vi "plot_radar_target_by_name.vi"(4 "error in":errorcluster={"status"=FALSE, "code"=0, "source"="Event Code: 0\r\ncomplete\r\n-----------------------------------\nEvent Code: 0\r\ncomplete\r\n-----------------------------------\nEvent Code: 0\r\nweather configured to \"Default\"\r\n-----------------------------------\nEvent Code: 0\r\ncomplete\r\n-----------------------------------\nEvent Code: 0\r\nsimulator configuration mode = 1\r\n-----------------------------------\nEvent Code: 0\r\nsimulator_version: 1.10.0, api_version: 3.0\r\n-----------------------------------\nEvent Code: 0\r\n\r\n-----------------------------------\n"}, 6 "Target id to track":string="compact_monoDrive_01_2", 7 "Radar Sample":T1={"Number of targets"=14, "gt_targets"=[], "target_list"=[{"aoa"=14.62, "range"=9.3, "rcs"=-11.41, "velocity"=-6.5, "target_ids"=["GuardRails14", "GuardRails13"]}, {"aoa"=-1.91, "range"=10.92, "rcs"=-12.49, "velocity"=-6.62, "target_ids"=[]}, {"aoa"=-1.49, "range"=12.13, "rcs"=-17.08, "velocity"=-6.5699997, "target_ids"=["truck_monoDrive_01_2"]}, {"aoa"=10.91, "range"=13.75, "rcs"=-16.51, "velocity"=-6.6499996, "target_ids"=["GuardRails14"]}, {"aoa"=9.55, "range"=14.549999, "rcs"=-14.82, "velocity"=-6.6499996, "target_ids"=["GuardRails14"]}, {"aoa"=8.45, "range"=16.17, "rcs"=-14.36, "velocity"=-6.64, "target_ids"=["GuardRails14"]}, {"aoa"=8.429999, "range"=17.789999, "rcs"=-10.95, "velocity"=-6.6499996, "target_ids"=["GuardRails14"]}, {"aoa"=6.6499996, "range"=20.21, "rcs"=-9.48, "velocity"=-6.64, "target_ids"=["GuardRails14"]}, {"aoa"=6.33, "range"=24.26, "rcs"=-13.74, "velocity"=-6.64, "target_ids"=["GuardRails15"]}, {"aoa"=13.61, "range"=27.09, "rcs"=-7.4199996, "velocity"=-6.6499996, "target_ids"=["InstancedFoliageActor_0"]}, {"aoa"=4.69, "range"=31.539999, "rcs"=-13.62, "velocity"=-6.64, "target_ids"=["GuardRails15"]}, {"aoa"=4.2999997, "range"=35.17, "rcs"=-11.82, "velocity"=-6.64, "target_ids"=["GuardRails15"]}, {"aoa"=-12.49, "range"=52.559998, "rcs"=12.82, "velocity"=-6.6499996, "target_ids"=["prp_electricalBox_142"]}, {"aoa"=-11.08, "range"=52.559998, "rcs"=12.82, "velocity"=-6.6499996, "target_ids"=["HighwaySign_30"]}], "tracks"=[], "roi_targets"=[]}) -> (0 "error out":errorcluster={"status"=FALSE, "code"=0, "source"="Event Code: 0\r\ncomplete\r\n-----------------------------------\nEvent Code: 0\r\ncomplete\r\n-----------------------------------\nEvent Code: 0\r\nweather configured to \"Default\"\r\n-----------------------------------\nEvent Code: 0\r\ncomplete\r\n-----------------------------------\nEvent Code: 0\r\nsimulator configuration mode = 1\r\n-----------------------------------\nEvent Code: 0\r\nsimulator_version: 1.10.0, api_version: 3.0\r\n-----------------------------------\nEvent Code: 0\r\n\r\n-----------------------------------\n"})   [LabVIEW 2019, in "Lib_Simx.lvlib"]
doc: "Tool generates a plot to compare AoA, Range and Velocity between the GT targets and the target list from the Radar sensor. This tool only tracks one target by the specified target on the Name of Target control."
uses:
  Lib_Simx.lvlib
  controls/radarSample.ctl
  controls/RadarTrack.ctl
panel:
  out "Velocity":cluster{"t":sgl, "t":sgl}(graph)
  out "Range":cluster{"t":sgl, "t":sgl}(graph)
  out "Aoa":cluster{"t":sgl, "t":sgl}(graph)
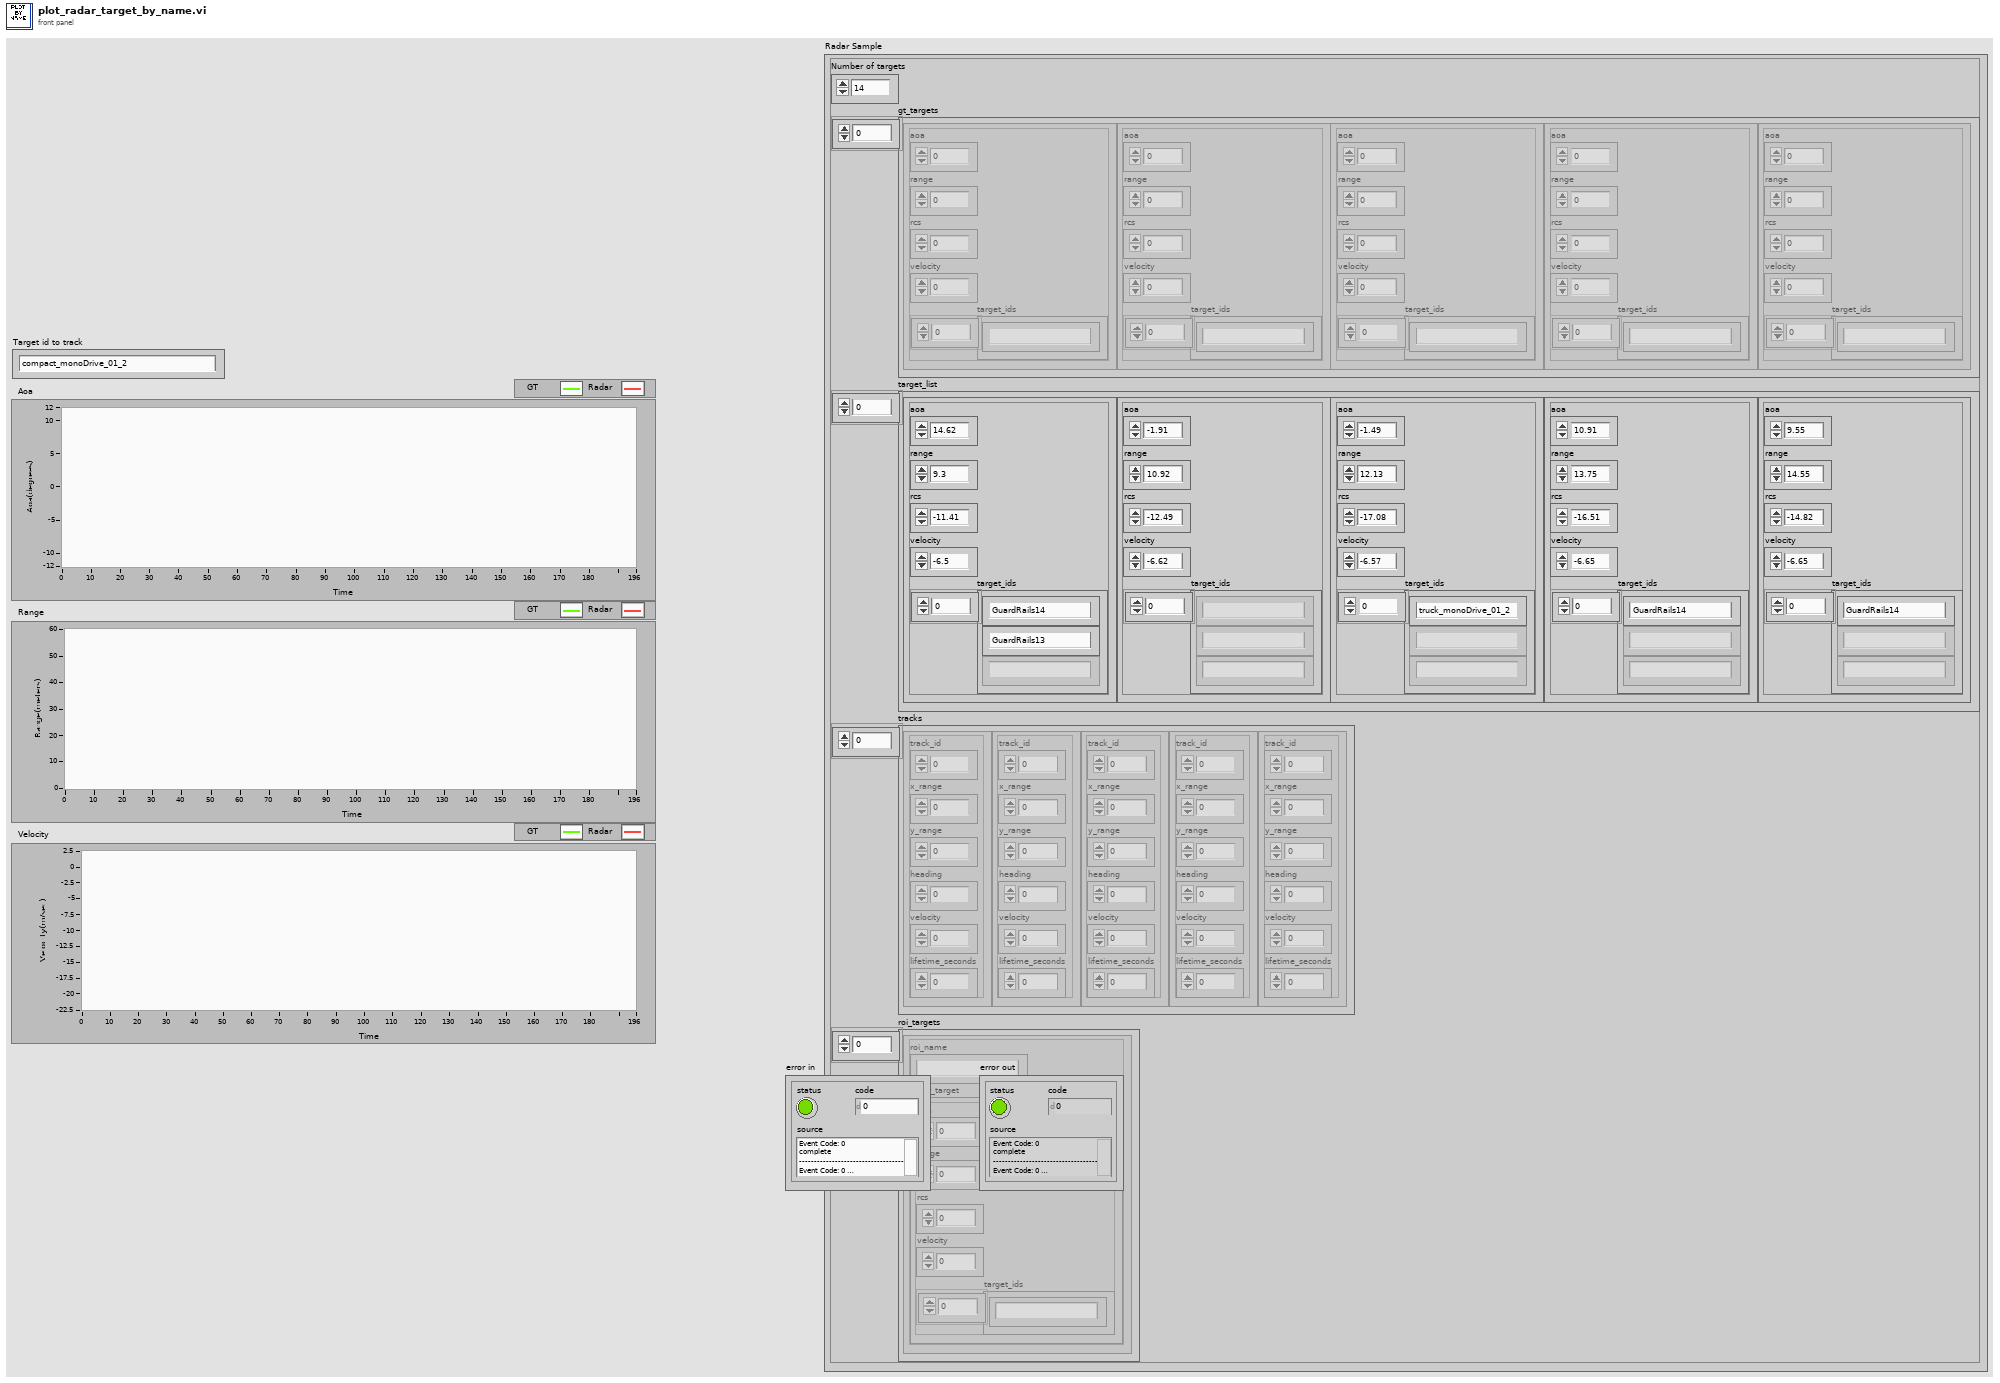
[diagram p1: front panel]
types:
  T1 = typedef "Lib_Simx.lvlib/radarSample.ctl" = cluster{"Number of targets":i32, "gt_targets":cluster{"aoa":sgl, "range":sgl, "rcs":sgl, "velocity":sgl, "target_ids":string[]}[], "target_list":cluster{"aoa":sgl, "range":sgl, "rcs":sgl, "velocity":sgl, "target_ids":string[]}[], "tracks":T2[], "roi_targets":cluster{"roi_name":string, "radar_target":cluster{"aoa":sgl, "range":sgl, "rcs":sgl, "velocity":sgl, "target_ids":string[]}}[]}
  T2 = typedef "Lib_Simx.lvlib/RadarTrack.ctl" = cluster{"track_id":u64, "x_range":sgl, "y_range":sgl, "heading":sgl, "velocity":sgl, "lifetime_seconds":sgl}
  T3 = cluster{"aoa":sgl, "range":sgl, "rcs":sgl, "velocity":sgl, "target_ids":string[]}[]
  T4 = cluster{"Average Range":sgl, "Average Range":sgl}
  T5 = cluster{"Average Velocity":sgl, "Average Velocity":sgl}
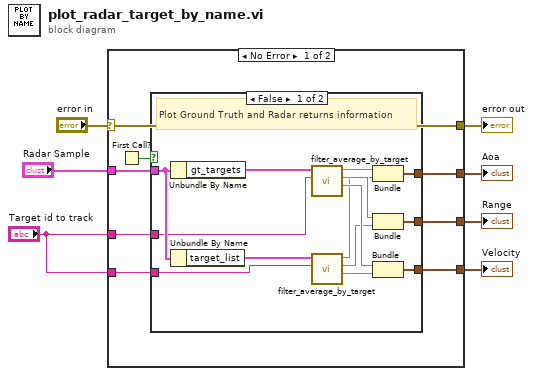
[diagram p0: block diagram]
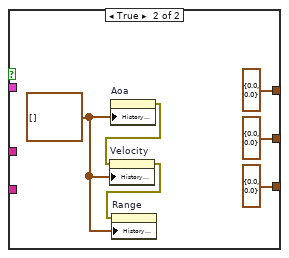
[diagram p2: hidden frame]
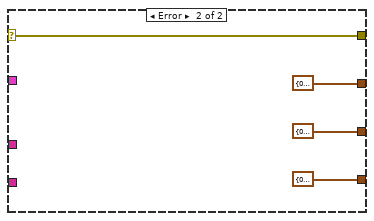
[diagram p3: hidden frame]
diagram:
  n1 = case shown="No Error" "error in" {
    selector: "error in" -> [w10 w39]
    tunnel: [w10 w39] -> w7
    tunnel: "Radar Sample" -> [w15 _]
    tunnel: [w14 cluster{"t":sgl, "t":sgl} {"t"=0.0, "t"=0.0}] -> w5
    tunnel: [w13 cluster{"t":sgl, "t":sgl} {"t"=0.0, "t"=0.0}] -> w4
    tunnel: [w12 cluster{"t":sgl, "t":sgl} {"t"=0.0, "t"=0.0}] -> w3
    tunnel: "Target id to track" -> [w9 _]
    tunnel: "Target id to track" -> [w8 _]
    frame No Error {
      n2 = First Call?() -> (First Call?: T/F=w11:bool)
      n3 = case shown="False" w11 {
        tunnel: w15 -> [w29 _]
        tunnel: [w27 cluster{"Average AoA":sgl, "Average AoA":sgl} {"Average AoA"=0.0, "Average AoA"=0.0}] -> w14
        tunnel: [w26 cluster{"Average AoA":sgl, "Average AoA":sgl} {"Average AoA"=0.0, "Average AoA"=0.0}] -> w13
        tunnel: [w22 cluster{"Average AoA":sgl, "Average AoA":sgl} {"Average AoA"=0.0, "Average AoA"=0.0}] -> w12
        tunnel: w9 -> [w17 _]
        tunnel: w8 -> [w16 _]
        frame False {
          # "Plot Ground Truth and Radar returns information"
          n4 = Unbundle By Name(w29) -> ("gt_targets"=w28:T3)
          n5 = Unbundle By Name(w29) -> ("target_list"=w21:T3)
          n6 = call "filter_average_by_target.vi"("Target id to track"=w16, "Targets"=w28) -> ("Average Velocity"=w25:sgl, "Average Range"=w24:sgl, "Average AoA"=w23:sgl)  [unwired: 3 in]
          n7 = call "filter_average_by_target.vi"("Target id to track"=w17, "Targets"=w21) -> ("Average Velocity"=w18:sgl, "Average Range"=w19:sgl, "Average AoA"=w20:sgl)  [unwired: 3 in]
          n8 = Bundle("Average AoA"=w23, "Average AoA"=w20) -> (w27:cluster{"Average AoA":sgl, "Average AoA":sgl})  [unwired: 1 in]
          n9 = Bundle("Average Range"=w24, "Average Range"=w19) -> (w26:T4)  [unwired: 1 in]
          n10 = Bundle("Average Velocity"=w25, "Average Velocity"=w18) -> (w22:T5)  [unwired: 1 in]
        }
        frame True {
          w30 = cluster{"t":sgl, "t":sgl}[] [] ("History Data")
          n11 = property on="Aoa" class="WFChart (strict)"("History Data"=w30) -> (error out=w32:errorcluster)  [unwired: 2 in, 1 out]
          n12 = property on="Velocity" class="WFChart (strict)"(error in=w32, "History Data"=w30) -> (error out=w31:errorcluster)  [unwired: 1 in, 1 out]
          n13 = property on="Range" class="WFChart (strict)"(error in=w31, "History Data"=w30) -> ()  [unwired: 1 in, 2 out]
        }
      }
    }
    frame Error {
    }
  }
  "error out" <- w7
  "Aoa" <- w5
  "Velocity" <- w3
  "Range" <- w4
